vi "plot_pressure_time_dependance_range.vi"() -> ()   [LabVIEW 2019]
panel:
  out "error out":errorcluster
  in  "End scan time / s":dbl
  in  "Valve Close Time / s":dbl
  in  "Valve Open Time / s":dbl
  in  "Backing Pressure / Bar":dbl format="%#_13g"
  in  "Gas Type":string="flow_pressure_calibration"
  in  "Lower bound":dbl=4e-06
  in  "Step size":dbl=5e-07
  in  "Upper bound":dbl=5e-05
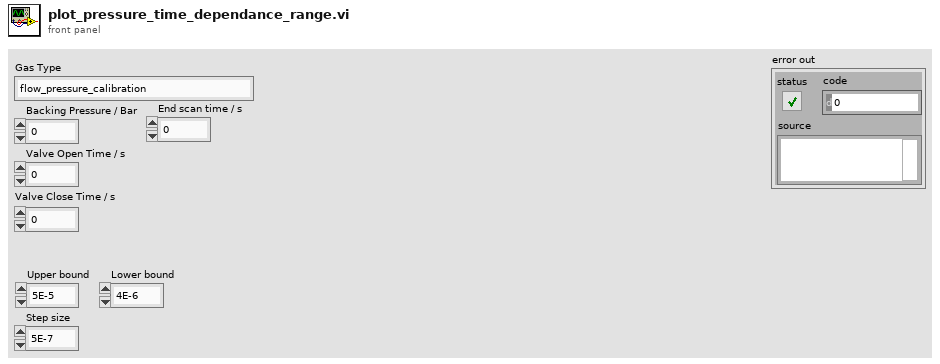
[diagram p1: front panel]
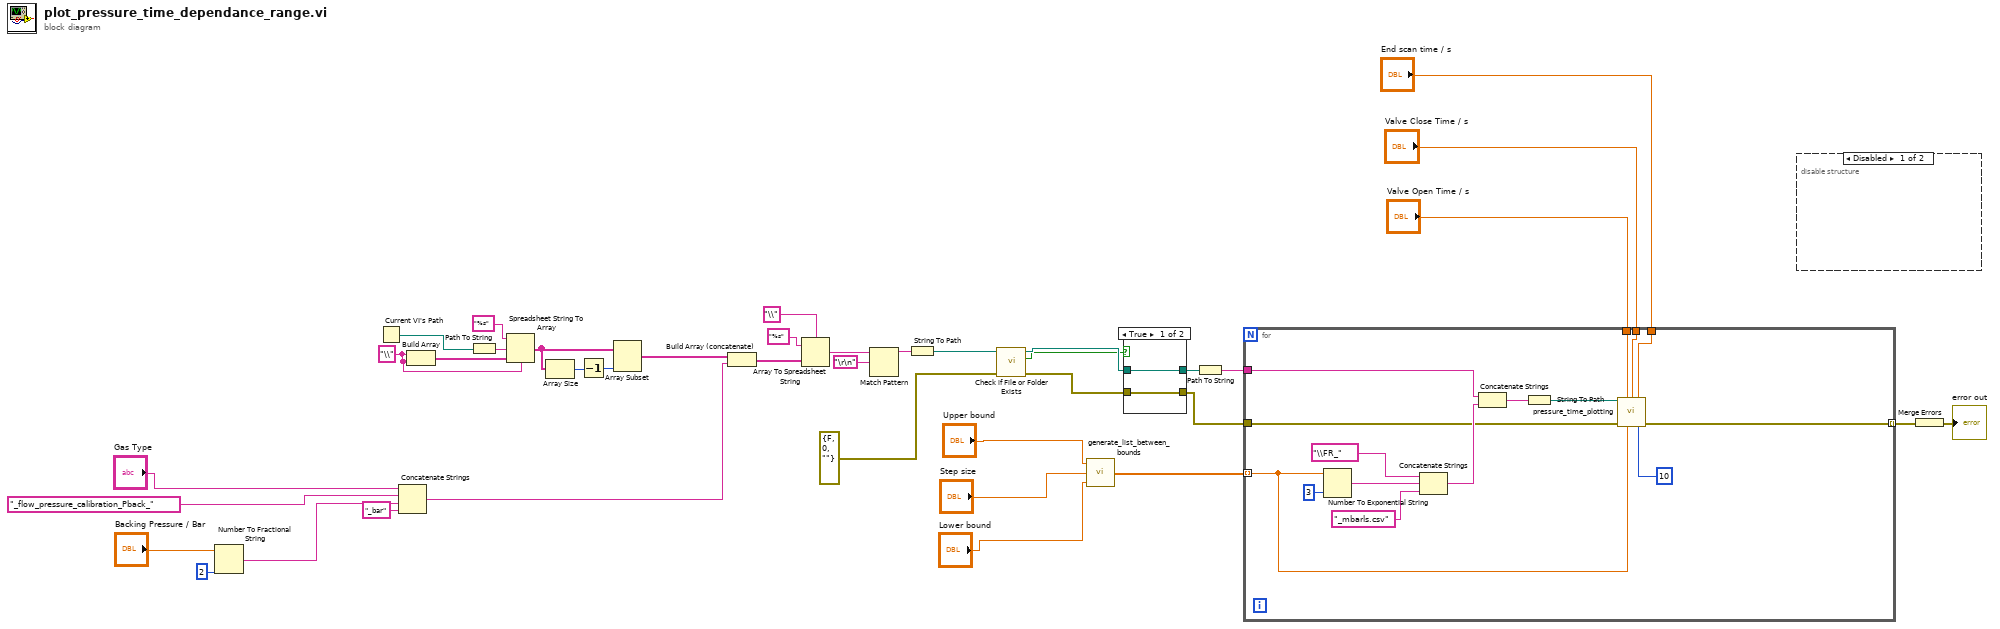
[diagram p0: block diagram]
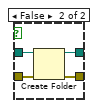
[diagram p2: hidden frame]
diagram:
  w31 = "\\" ("delimiter (Tab)")
  n1 = Number To Fractional String(number="Backing Pressure / Bar", precision (6)=i16 2) -> (F-format string=w35:string)  [unwired: 2 in]
  n2 = Current VI's Path() -> (path=w15:path)
  n3 = Concatenate Strings("Gas Type", "_flow_pressure_calibration_Pback_", w35, "_bar" ("string")) -> (w12:string)
  n4 = Build Array(w31, w31) -> (w30:string[])
  n5 = Path To String(path=w15) -> (string=w32:string)
  n6 = Spreadsheet String To Array(delimiter (Tab)=w31, format string="%s", spreadsheet string=w32, array type (2D Dbl)=w30) -> (array=w28:string[])
  n7 = Array Size(array=w28) -> (size(s)=w24:i32)
  n8 = Decrement(x=w24) -> (x-1=w27:i32)
  n9 = Array Subset(array=w28, length=w27) -> (w23:string[])  [unwired: 1 in]
  n10 = Build Array (concatenate)(w23, w12) -> (w22:string[])
  n11 = Array To Spreadsheet String(delimiter (Tab)="\\", array=w22, 3:"%s" ("format string")) -> (spreadsheet string=w21:string)
  n12 = Match Pattern(string=w21, regular expression="\r\n") -> (before substring=w20:string)  [unwired: 1 in, 3 out]
  n13 = String To Path(string=w20) -> (path=w18:path)
  n14 = call <vilib>:"Check if File or Folder Exists.vi"("error in (no error)"=errorcluster {"status"=FALSE, "code"=0, "source"=""}, "path"=w18) -> ("error out"=w11:errorcluster, "file or folder exists?"=w16:bool, "dup path"=w17:path)  [unwired: 7 in]
  n15 = call "generate_list_between_bounds.vi"("Upper bound"="Upper bound", "Step size"="Step size", "Lower bound"="Lower bound") -> ("Array"=w33:dbl[])  [unwired: 2 in]
  n16 = case shown="True" w16 {
    tunnel: w17 -> [w41 w45]
    tunnel: [w41 w44] -> w14
    tunnel: w11 -> [w40 w43]
    tunnel: [w40 w42] -> w9
    frame True {
    }
    frame False {
      n17 = Create Folder(path (use dialog)=w45, error in=w43) -> (created path=w44:path, error out=w42:errorcluster)  [unwired: 1 in, 1 out]
    }
  }
  n18 = Path To String(path=w14) -> (string=w13:string)
  n19 = for {
    tunnel: w33 -> [w52] mode=indexing
    tunnel: w13 -> [w55]
    tunnel: w9 -> [w51]
    tunnel: "Valve Open Time / s" -> [w50]
    tunnel: "Valve Close Time / s" -> [w49]
    tunnel: "End scan time / s" -> [w47]
    tunnel: [w46] -> w5 mode=indexing
    n20 = Number To Exponential String(number=w52, precision (6)=i16 3) -> (E-format string=w58:string)  [unwired: 2 in]
    n21 = Concatenate Strings("\\FR_", w58, "_mbarls.csv" ("string")) -> (w56:string)
    n22 = Concatenate Strings(w55, w56) -> (w54:string)
    n23 = String To Path(string=w54) -> (path=w53:path)
    n24 = call "pressure_time_plotting.vi"("file path (use dialog)"=w53, "Valve Open Time / s"=w50, "Valve Close Time / s"=w49, "End scan time / s"=w47, "error in (no error)"=w51, "Set Flow / mbar ls-1"=w52, "Target Recording Frequency / Hz"=10) -> ("error out"=w46:errorcluster)  [unwired: 8 in]
  }
  n25 = disable-structure shown="Disabled" {
    frame Disabled {
    }
    frame Enabled {
    }
  }
  n26 = Merge Errors(w5) -> (→"error out":errorcluster)
